vi "Telnet Wait on Listener.vi"(8 "error in (no error)":errorcluster, 9 "timeout ms (wait forever : -1)":i32=-1, 11 "listener ID":refnum<k5>) -> (0 "error out":errorcluster, 1 "remote port":u16, 2 "remote address":string, 3 "listener ID out":refnum<k5>, 4 "telnet connection":T1)   [LabVIEW 2011]
uses:
  Telnet Session.ctl
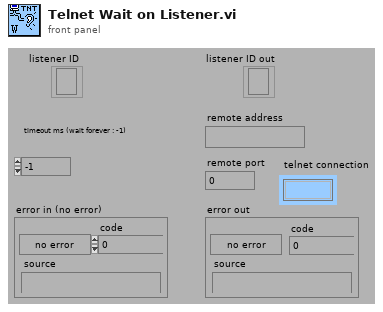
[diagram p1: front panel]
types:
  T1 = typedef "Telnet Session.ctl" = refnum<k1>
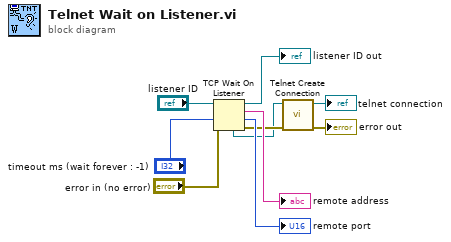
[diagram p0: block diagram]
diagram:
  n1 = TCP Wait On Listener(8:"error in (no error)", 9:"timeout ms (wait forever : -1)", 11:"listener ID") -> (0:w4:errorcluster, 1:→"remote port":u16, 2:→"remote address":string, 3:→"listener ID out":refnum<k5>, 4:w3:refnum<k5>)  [unwired: 1 in]
  n2 = call "Telnet Create Connection.vi"("error in (no error)"=w4, "TCP connection"=w3) -> ("error out"=→"error out":errorcluster, "telnet connection"=→"telnet connection":T1)  [unwired: 8 in]
